vi "cluster_calculation.vi"() -> ()   [LabVIEW 2021]
panel:
  out "length":cluster{"name":i32, "email":i32}
  out "x+y":cluster{"x":dbl, "y":dbl}
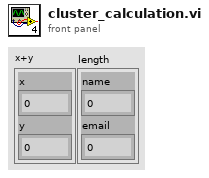
[diagram p1: front panel]
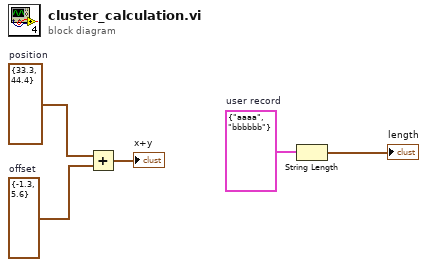
[diagram p0: block diagram]
diagram:
  w2 = cluster{"name":string, "email":string} {"name"="aaaa", "email"="bbbbbb"}  # user record
  w4 = cluster{"x":dbl, "y":dbl} {"x"=-1.3, "y"=5.6}  # offset
  w5 = cluster{"x":dbl, "y":dbl} {"x"=33.3, "y"=44.4}  # position
  n1 = Add(x=w5, y=w4) -> (x+y=→"x+y":cluster{"x":dbl, "y":dbl})
  n2 = String Length(string=w2) -> (length=→"length":cluster{"name":i32, "email":i32})
